vi "Get Connection Reference.vi"(8 "error in (no error)":errorcluster, 11 "SQLite3LV Connection in":refnum<class "sqlite3.lvclass">) -> (0 "error out":errorcluster, 2 "ppDb":i64 format="%.0x", 3 "SQLite3LV Connection out":refnum<class "sqlite3.lvclass">)   [LabVIEW 2014, in "SQLite3LV.lvlib" / "sqlite3.lvclass"]
uses:
  sqlite3.lvclass
  sqlite3.lvclass/sqlite3.ctl
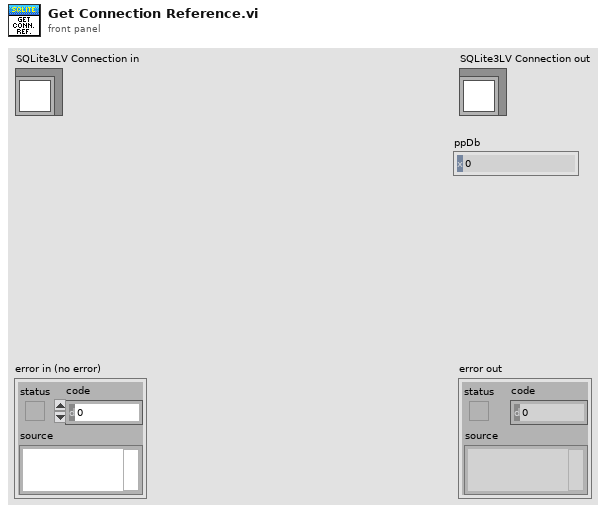
[diagram p1: front panel]
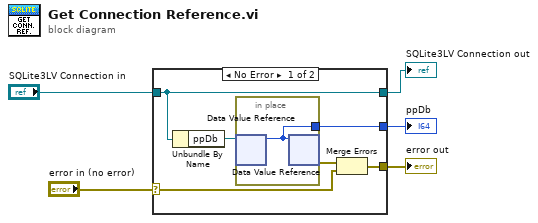
[diagram p0: block diagram]
diagram:
  n1 = case shown="No Error" "error in (no error)" {
    selector: "error in (no error)" -> [w7 w14]
    tunnel: [w6 w14] -> w4
    tunnel: [w11 w13] -> w2
    tunnel: "SQLite3LV Connection in" -> [w11 w13]
    tunnel: [w9 _] -> w1
    frame No Error {
      n2 = Unbundle By Name(w11) -> ("ppDb"=w10:refnum<data-value>)
      n3 = in-place {
        in-place-border: [w12] -> w9
        n4 = in-place-dvr #1(w10) -> (w12:i64)  [unwired: 1 out]
        n5 = in-place-dvr #1(w12) -> (w8:errorcluster)  [unwired: 1 out]
      }
      n6 = Merge Errors(w8, w7) -> (w6:errorcluster)
    }
    frame Error {
    }
  }
  "error out" <- w4
  "SQLite3LV Connection out" <- w2
  "ppDb" <- w1
